vi "SCD - load LCVR Voltages.vi"(3 "input rcp":dbl[](array[numeric])=[1.8374212607235123, 1.6766025168197034, 2.2097290599219055, 2.2205289350684585, 1.959581474179891] format="%.4f") -> (1 "Required LCVR Voltages":dbl[](array[numeric])=[1.8374212607235123, 1.6766025168197034, 2.2097290599219055, 2.2205289350684585, 1.959581474179891] format="%.4f")   [LabVIEW 2014]
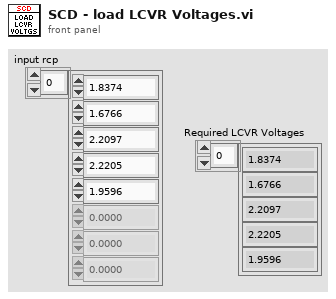
[diagram p1: front panel]
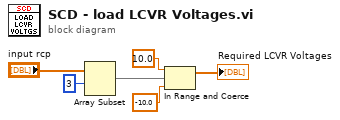
[diagram p0: block diagram]
diagram:
  n1 = Array Subset(array="input rcp", index=3) -> (w1:dbl[])  [unwired: 1 in]
  n2 = In Range and Coerce(upper limit=10.0, x=w1, lower limit=-10.0) -> (coerced(x)=→"Required LCVR Voltages":dbl[])  [unwired: 1 out]
